vi "cleanup.vi"(0 "handle":u32, 11 "error in (no error)":errorcluster) -> (2 "function return":i32, 15 "error out":errorcluster)   [LabVIEW 2013, in "buddy.lvlib"]
doc: "EXPORT int buddy_cleanup(hid_device *handle, buddy_hid_info_t *hid_info);"
uses:
  buddy.lvlib
  buddy/x64/Debug/buddy.dll
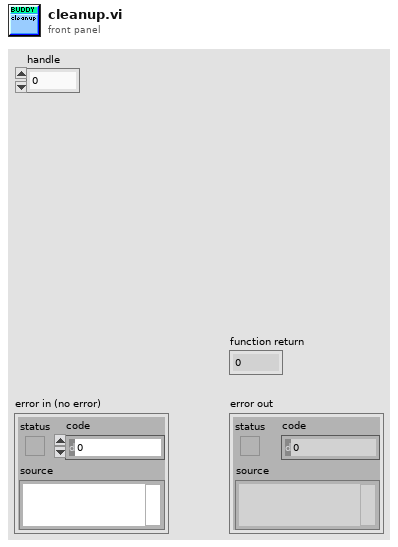
[diagram p1: front panel]
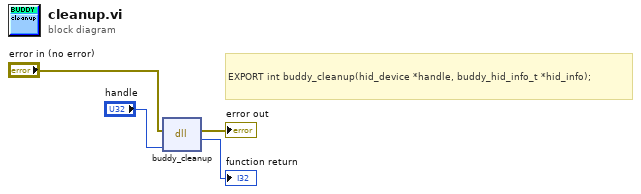
[diagram p0: block diagram]
diagram:
  # "EXPORT int buddy_cleanup(hid_device *handle, buddy_hid_info_t *hid_info);"
  n1 = dll-call lib="C:/Users/shraken/shraken_code/usbhid_buddy/lib/libbuddy/bindings/labview/buddy/x64/Debug/buddy.*" fn="buddy_cleanup"(error in="error in (no error)", "handle"="handle") -> (error out=→"error out":errorcluster, "return type"=→"function return":i32)  [unwired: 3 in, 1 out]
